vi "Import SystemLink State Example.vi"() -> ()   [LabVIEW 2017]
uses:
  SystemLink_States_API.lvlib
panel:
  out "error out":errorcluster
  out "state metadata":string
  in  "state description":string
  in  "state filepath":path
  in  "state name":string
  in  "password":string
  in  "username":string
  in  "SystemLink server base URL":string="https://"
  # "SystemLink Server"
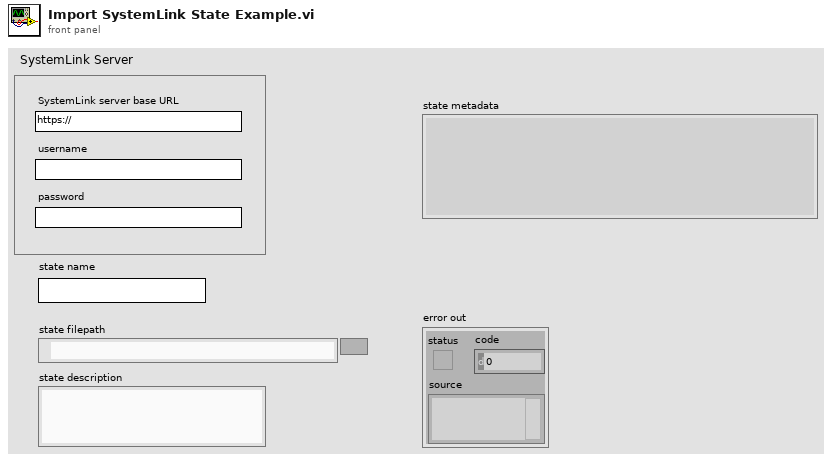
[diagram p1: front panel]
types:
  T1 = typedef "SystemLink_States_API.lvlib/systemlink connection.ctl" = cluster{"client handle out":T2, "SystemLink server base URL":string}
  T2 = typedef "LabVIEWHTTPClient.lvlib/ClientHandle.ctl" = refnum<k1>
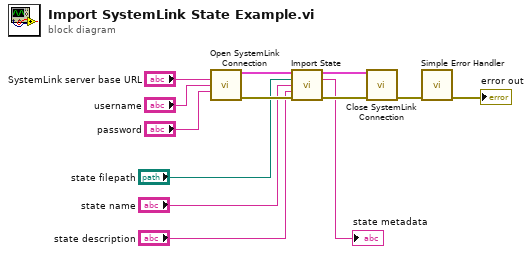
[diagram p0: block diagram]
diagram:
  n1 = call "Open SystemLink Connection.vi"("SystemLink server base URL"="SystemLink server base URL", "username"="username", "password"="password") -> ("SystemLink connection out"=w9:T1, "error out"=w7:errorcluster)  [unwired: 11 in]
  n2 = call "Import State.vi"("SystemLink connection in"=w9, "state filepath"="state filepath", "state name"="state name", "state description"="state description", "error in (no error)"=w7) -> ("SystemLink connection out"=w8:T1, "state metadata"=→"state metadata":string, "error out"=w6:errorcluster)  [unwired: 8 in]
  n3 = call "Close SystemLink Connection.vi"("SystemLink connection in"=w8, "error in (no error)"=w6) -> ("error out"=w10:errorcluster)  [unwired: 13 in]
  n4 = call <vilib>:"Simple Error Handler.vi"("error in (no error)"=w10) -> ("error out"=→"error out":errorcluster)  [unwired: 4 in, 4 out]
